vi "Get COM by Descriptor.vi"(8 "error in (no error)":errorcluster, 10 "Generate error if no COM port found? (False)":bool, 11 "COM descriptor":string) -> (0 "error out":errorcluster, 1 "First COM port":T1, 2 "COM ports count":i32, 3 "COM list":T1[](array[typedef]))   [LabVIEW 2020, in "Get COM Descriptor.lvlib"]
doc: "Get list of COM ports matching given descriptor.\n\nDetails: https://github.com/smaslan/get-com-descriptor"
uses:
  Get COM Descriptor.lvlib
  COM port.ctl
  <vilib>/Utility/error.llb/Error Cluster From Error Code.vi
  <vilib>/ErrorRing/Error Ring.xnode
  get_com_descriptor.dll
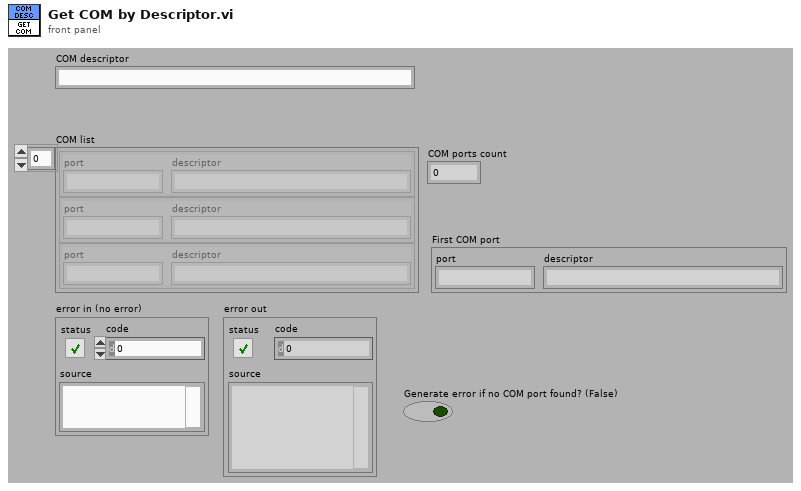
[diagram p1: front panel]
types:
  T1 = typedef "Get COM Descriptor.lvlib/COM port.ctl" = cluster{"port":string, "descriptor":string}
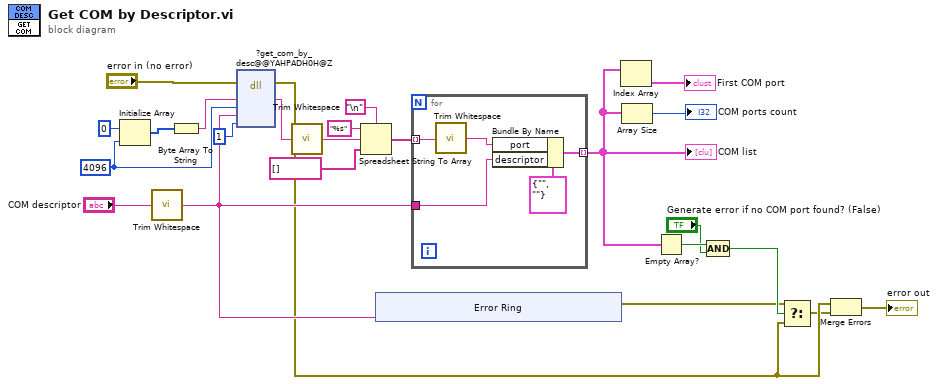
[diagram p0: block diagram]
diagram:
  w20 = 4096 ("dimension size")
  n1 = Initialize Array(u8 0 ("element"), w20) -> (w23:u8[])
  n2 = call <vilib>:"Trim Whitespace.vi"("string"="COM descriptor") -> ("trimmed string"=w10:string)  [unwired: 1 in]
  n3 = Byte Array To String(unsigned byte array=w23) -> (string=w21:string)
  n4 = dll-call lib="F:/Z_bridge_v4/other/get_com_descriptor/get_com_descriptor.dll" fn="?get_com_by_desc@@YAHPADH0H@Z"(error in="error in (no error)", "buf"=w21, "size"=w20, "desc"=w10, "to_ascii"=1) -> (error out=w4:errorcluster, "buf"=w19:string)  [unwired: 6 in, 1 out]
  n5 = call <vilib>:"Trim Whitespace.vi"("string"=w19) -> ("trimmed string"=w18:string)  [unwired: 1 in]
  n6 = Spreadsheet String To Array(delimiter (Tab)="\n", format string="%s", spreadsheet string=w18, array type (2D Dbl)=string[] []) -> (array=w15:string[])
  n7 = xnode "Error Ring"("parameter 0"=w10) -> ("error out"=w5:errorcluster)
  n8 = for {
    tunnel: w15 -> [w29] mode=indexing
    tunnel: [w27] -> w9 mode=indexing
    tunnel: w10 -> [w25]
    n9 = call <vilib>:"Trim Whitespace.vi"("string"=w29) -> ("trimmed string"=w26:string)  [unwired: 1 in]
    n10 = Bundle By Name(cluster=T1 {"port"="", "descriptor"=""} ("COM port"), "port"=w26, "descriptor"=w25) -> (w27:T1)
  }
  "COM list" <- w9
  n11 = Index Array(array=w9) -> (element=→"First COM port":T1)  [unwired: 1 in]
  n12 = Array Size(array=w9) -> (size(s)=→"COM ports count":i32)
  n13 = Empty Array?(array=w9) -> (empty?=w8:bool)
  n14 = Compound Arithmetic op=AND(w8, "Generate error if no COM port found? (False)") -> (w6:bool)
  n15 = Select(t=w5, s=w6, f=w4) -> (s? t:f=w3:errorcluster)
  n16 = Merge Errors(w4, w3) -> (→"error out":errorcluster)
